vi "PAC2INS.vi"(0 "PACKET":string) -> (1 "TYPE":T1(ring), 2 "SEQUENCE":u32, 3 "LENGTH":u32, 4 "BODY":u8[](array[numeric]))   [LabVIEW 2016]
panel:
  out "unsigned byte array":u8[](array[numeric]) format="%b"
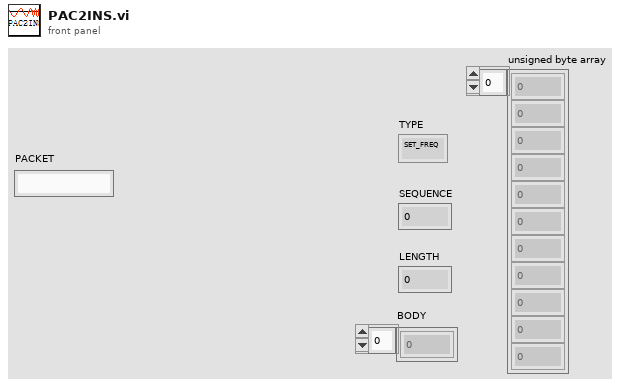
[diagram p1: front panel]
types:
  T1 = enum8{"SET_FREQ", "SET_VOLT", "SET_CHENNEL_VOLT", "SET_PHASE", "START_HEAT", "STOP_HEAT", "CHANNEL_CTRL_SINGLE", "CHANNEL_CTRL_ALL", "READ_VOLT_SET", "READ_VOLT_SET_RSP", "READ_CURRENT_VOLT", "READ_CURRENT_VOLT_RSP", "READ_PHASE", "READ_PHASE_RSP", "READ_HEATTIME_LEFT", "READ_HEATTIME_LEFT_RSP", "EXEC_RSP"}
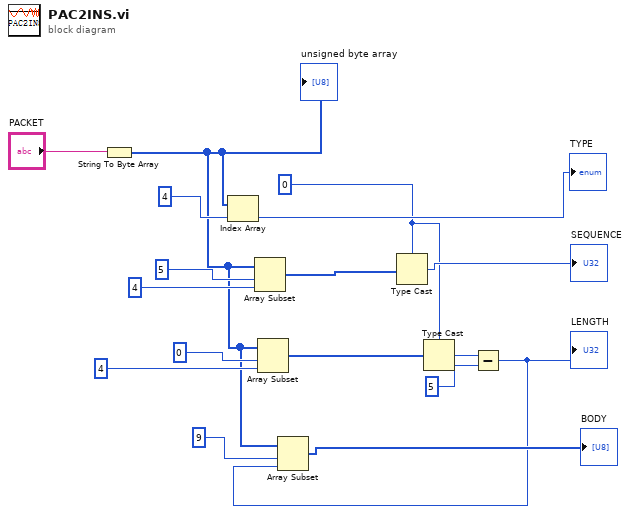
[diagram p0: block diagram]
diagram:
  w9 = u32 0
  n1 = String To Byte Array(string="PACKET") -> (unsigned byte array=w8:u8[])
  "unsigned byte array" <- w8
  n2 = Index Array(array=w8, index=4) -> (element=→"TYPE":u8)
  n3 = Array Subset(array=w8, index=5, length=4) -> (w4:u8[])
  n4 = Array Subset(array=w8, index=0, length=4) -> (w5:u8[])
  n5 = Type Cast(type=w9, x=w4) -> (*(type *) &x=→"SEQUENCE":u32)
  n6 = Type Cast(type=w9, x=w5) -> (*(type *) &x=w3:u32)
  n7 = Subtract(x=w3, y=u32 5) -> (x-y=w1:u32)
  "LENGTH" <- w1
  n8 = Array Subset(array=w8, index=9, length=w1) -> (→"BODY":u8[])
